vi "Read Namespace Symbol Information.vi"(8 "error in (no error)":errorcluster, 9 "Get all descendents?":bool, 10 "Namespace":string, 11 "TwinCAT ADS in":refnum<class "TwinCAT ADS.lvclass">) -> (0 "error out":errorcluster, 1 "Symbols Information":T1[](array[typedef]) {"Type ID" items=["ADST_VOID"=0, "ADST_INT16"=2, "ADST_INT32"=3, "ADST_REAL32"=4, "ADST_REAL64"=5, "ADST_INT8"=16, "ADST_UINT8"=17, "ADST_UINT16"=18, "ADST_UINT32"=19, "ADST_INT64"=20, "ADST_UINT64"=21, "ADST_STRING"=30, "ADST_WSTRING"=31, "ADST_REAL80"=32, "ADST_BIT"=33, "ADST_MAXTYPES"=34, "ADST_BIGTYPE"=65]; "Type Category" items=["Unknown, None"=0, "Primitive"=1, "Alias"=2, "Enum"=3, "Array"=4, "Struct"=5, "FunctionBlock"=6, "Program"=7, "Function"=8, "SubRange"=9, "String"=10, "Bitset"=12, "Pointer"=13, "Union"=14, "Reference"=15, "Interface"=16]}, 3 "TwinCAT ADS out":refnum<class "TwinCAT ADS.lvclass">)   [LabVIEW 2018, in "TwinCAT ADS.lvclass"]
uses:
  TwinCAT ADS.lvclass
  Controls/Symbol Information.ctl
  TwinCAT ADS.lvclass/TwinCAT ADS.ctl
  TwinCAT.Ads
  <vilib>/regexp/Match Regular Expression.xnode
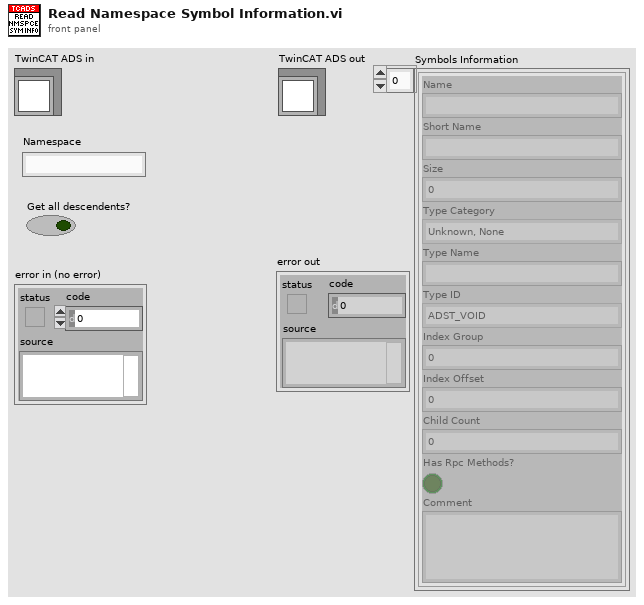
[diagram p1: front panel]
types:
  T1 = typedef "TwinCAT ADS.lvclass/Symbol Information.ctl" = cluster{"Name":string, "Short Name":string, "Size":i32, "Type Category":i32, "Type Name":string, "Type ID":i32, "Index Group":i64, "Index Offset":i64, "Child Count":i32, "Has Rpc Methods?":bool, "Comment":string}
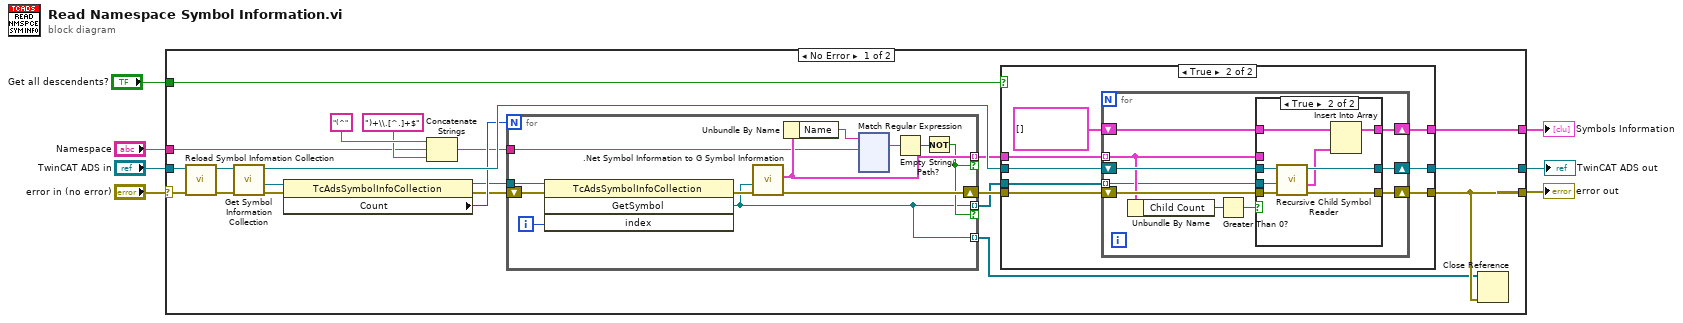
[diagram p0: block diagram]
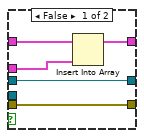
[diagram p3: hidden frame]
diagram:
  n1 = case shown="No Error" "error in (no error)" {
    selector: "error in (no error)" -> [w16 w191]
    tunnel: [w9 w191] -> w6
    tunnel: [w24 w190] -> w4
    tunnel: "TwinCAT ADS in" -> [w17 w190]
    tunnel: "Namespace" -> [w10 _]
    tunnel: [w22 _] -> w2
    tunnel: "Get all descendents?" -> [w21 _]
    frame No Error {
      n2 = call "Reload Symbol Infomation Collection.vi"("error in (no error)"=w16, "TwinCAT ADS in"=w17) -> ("error out"=w14:errorcluster, "TwinCAT ADS out"=w15:refnum<class "TwinCAT ADS.lvclass">)  [unwired: 8 in]
      n3 = call "Get Symbol Information Collection.vi"("error in (no error)"=w14, "TwinCAT ADS in"=w15) -> ("error out"=w19:errorcluster, ".NET AdsSymbolInfoCollection"=w18:refnum<k24>, "TwinCAT ADS out"=w29:refnum<class "TwinCAT ADS.lvclass">)  [unwired: 7 in]
      n4 = property class="TcAdsSymbolInfoCollection"(reference=w18, error in=w19) -> (reference out=w26:refnum<k24>, error out=w27:errorcluster, "Count"=w28:i32)
      n5 = Concatenate Strings("(^" ("format string"), w10, ")+\\.[^.]+$" ("string")) -> (w11:string)
      n6 = for {
        N: w28 -> [_]
        tunnel: w26 -> [w75]
        shift-right: [w71] -> w25
        shift-left: w27 -> [w73]
        tunnel: w11 -> [w66]
        tunnel: [w67] -> w23 mode=indexing if=w65
        tunnel: [w64] -> w20 mode=indexing if=w65
        tunnel: [w64] -> w8 mode=indexing
        i -> [w74]
        n7 = invoke class="TcAdsSymbolInfoCollection" method="GetSymbol"(reference=w75, error in=w73, "index"=w74) -> (error out=w72:errorcluster, "GetSymbol"=w64:refnum<k24>)  [unwired: 1 in, 2 out]
        n8 = call ".Net Symbol Information to G Symbol Information.vi"(".NET AdsSymbolInfo"=w64, "error in (no error)"=w72) -> ("Symbol Information"=w67:T1, "error out"=w71:errorcluster)  [unwired: 6 in, 1 out]
        n9 = Unbundle By Name(w67) -> ("Name"=w70:string)
        n10 = xnode "Match Regular Expression"("input string"=w70, "regular expression"=w66) -> ("whole match"=w68:string)  [unwired: 4 in, 4 out]
        n11 = Empty String/Path?(string/path=w68) -> (empty?=w69:bool)
        n12 = Not(x=w69) -> (.not. x?=w65:bool)
      }
      n13 = case shown="True" w21 {
        tunnel: w25 -> [w32 w40]
        tunnel: [w32 w39] -> w9
        tunnel: [w30 w38] -> w24
        tunnel: w29 -> [w30 w37]
        tunnel: w23 -> [w31 w36]
        tunnel: [w31 w35] -> w22
        tunnel: w20 -> [_ w33]
        frame False {
        }
        frame True {
          n14 = for {
            shift-right: [w50] -> w39
            shift-left: w40 -> [w44]
            shift-right: [w49] -> w38
            shift-left: w37 -> [w48]
            tunnel: w36 -> [w42] mode=indexing
            shift-right: [w45] -> w35
            shift-left: T1[] [] -> [w46]
            tunnel: w33 -> [w41] mode=indexing
            n15 = Unbundle By Name(w42) -> ("Child Count"=w43:i32)
            n16 = Greater Than 0?(x=w43) -> (x > 0?=w47:bool)
            n17 = case shown="True" w47 {
              tunnel: w44 -> [w55 w61]
              tunnel: [w55 w57] -> w50
              tunnel: [w54 w58] -> w49
              tunnel: w48 -> [w54 w59]
              tunnel: w42 -> [w51 _]
              tunnel: w46 -> [w53 w63]
              tunnel: [w52 w62] -> w45
              tunnel: w41 -> [_ w60]
              frame False {
                n18 = Insert Into Array(array=w53, new element=w51) -> (w52:T1[])  [unwired: 1 in]
              }
              frame True {
                n19 = call "Recursive Child Symbol Reader.vi"("error in (no error)"=w61, ".NET TcAdsSymbolInfo"=w60, "TwinCAT ADS in"=w59) -> ("error out"=w57:errorcluster, "Symbols Information"=w56:T1[], "TwinCAT ADS out"=w58:refnum<class "TwinCAT ADS.lvclass">)  [unwired: 6 in]
                n20 = Insert Into Array(array=w63, new element=w56) -> (w62:T1[])  [unwired: 1 in]
              }
            }
          }
        }
      }
      n21 = Close Reference(reference=w8, error in (no error)=w9) -> ()  [unwired: 1 out]
    }
    frame Error {
    }
  }
  "error out" <- w6
  "TwinCAT ADS out" <- w4
  "Symbols Information" <- w2
